vi "LEP_RV_MsgBox.vi"(8 "Message":string, 11 "µVision":string="µVision") -> ()   [LabVIEW 2011]
doc: "Displays <B>Error Message</B> and <B>Error Output</B> in the <B>Failed to build executable</B> dialog box."
panel:
  out "Text":string
  in  "ok":bool
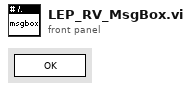
[diagram p1: front panel]
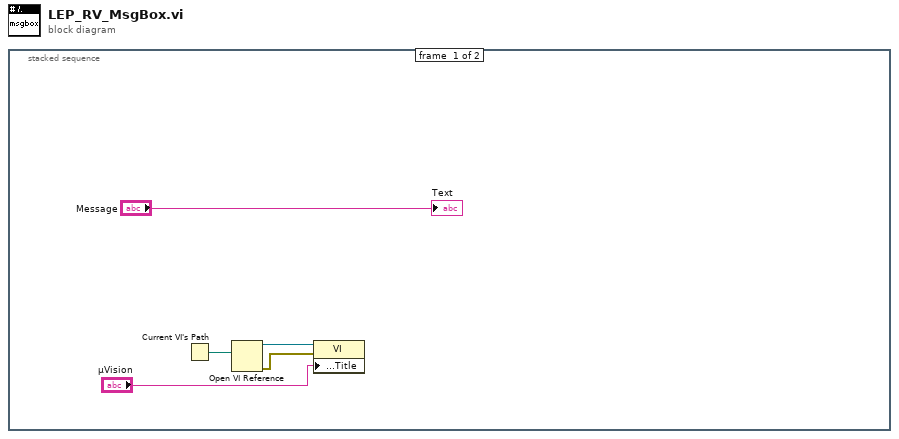
[diagram p0: block diagram]
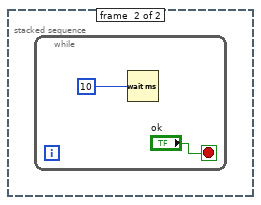
[diagram p2: hidden frame]
diagram:
  n1 = stacked-sequence {
    frame #0 {
      n2 = Current VI's Path() -> (path=w5:path)
      n3 = Open VI Reference(vi path=w5) -> (vi reference=w4:refnum<vi>, error out=w3:errorcluster)  [unwired: 5 in]
      n4 = property class="VI"(reference=w4, error in=w3, "Front Panel.Title"="µVision") -> ()  [unwired: 2 out]
      "Text" <- "Message"
    }
    frame #1 {
      n5 = while {
        stop <- "ok" stop-if-true
        n6 = Wait (ms)(milliseconds to wait=u32 10) -> ()  [unwired: 1 out]
      }
    }
  }
